vi "TC0608_Init.vi"(0 "object in":refnum<class "TC0608.lvclass">, 2 "VISA resource name":refnum<visa-resource-name>, 5 "error in (no error)":errorcluster) -> (14 "object out":refnum<class "TC0608.lvclass">, 19 "error out":errorcluster)   [LabVIEW 2023, in "TC0608.lvclass"]
uses:
  TC0608.lvclass
  TC0608.lvclass/TC0608.ctl
  Peltier controller TC/TCxxxx/TCxxxx.lvlib
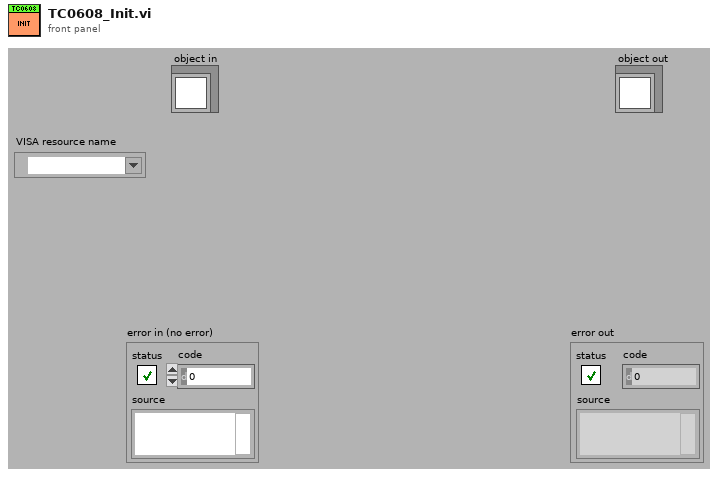
[diagram p1: front panel]
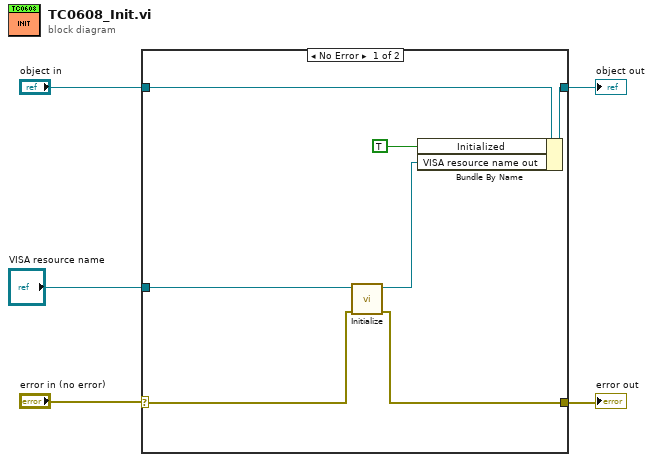
[diagram p0: block diagram]
diagram:
  n1 = case shown="No Error" "error in (no error)" {
    selector: "error in (no error)" -> [w8 w13]
    tunnel: "object in" -> [w12 w14]
    tunnel: [w11 w14] -> w4
    tunnel: [w7 w13] -> w2
    tunnel: "VISA resource name" -> [w9 _]
    frame No Error {
      n2 = call "Initialize.vi"("error in (no error)"=w8, "VISA resource name"=w9) -> ("error out"=w7:errorcluster, "VISA resource name out"=w6:refnum<visa-resource-name>)  [unwired: 8 in]
      n3 = Bundle By Name(cluster=w12, "Initialized"=TRUE ("None"), "VISA resource name out"=w6) -> (w11:refnum<class "TC0608.lvclass">)
    }
    frame Error {
    }
  }
  "object out" <- w4
  "error out" <- w2
